vi "DefendAreaTacticVSS.vi"(7 "First call?":bool=TRUE, 8 "error in (no error)":errorcluster, 9 "Game in":refnum<class "Game.lvclass">, 10 "Robot":refnum<class "Robot.lvclass">, 11 "DefendAreaTacticVSS in":refnum<class "DefendAreaTacticVSS.lvclass">) -> (0 "error out":errorcluster, 2 "Robot out":refnum<class "Robot.lvclass">, 3 "DefendAreaTacticVSS out":refnum<class "DefendAreaTacticVSS.lvclass">)   [LabVIEW 2020, in "DefendAreaTacticVSS.lvclass"]
uses:
  DefendAreaTacticVSS.lvclass
  Robot_class/Robot.lvclass
  Game_class/Game.lvclass
  Robot_class/tactics.ctl
  Tactic_class/Tactic.lvclass/Tactic.ctl
  Robot_class/Robot.lvclass/Robot.ctl
  Tactic_class/Read Skillbook.vi
  Robot_class/Write tactic.vi
  Skillbook_class/Skillbook.lvclass
  KickSkillVSS_class/KickSkillVSS.lvclass
  PenaltyPosSkillVSS_class/PenaltyPosSkillVSS.lvclass
  BallDispPosSkillVSS_class/BallDispPosSkillVSS.lvclass
  BallToGoalSkillVSS_class/BallToGoalSkillVSS.lvclass
  GoToBallSkillVSS_class/GoToBallSkillVSS.lvclass
  DefBallPosSkillVSS_class/DefBallPosSkillVSS.lvclass
  HaltSkill_class/HaltSkill.lvclass
panel:
  out "x .or. y?":bool
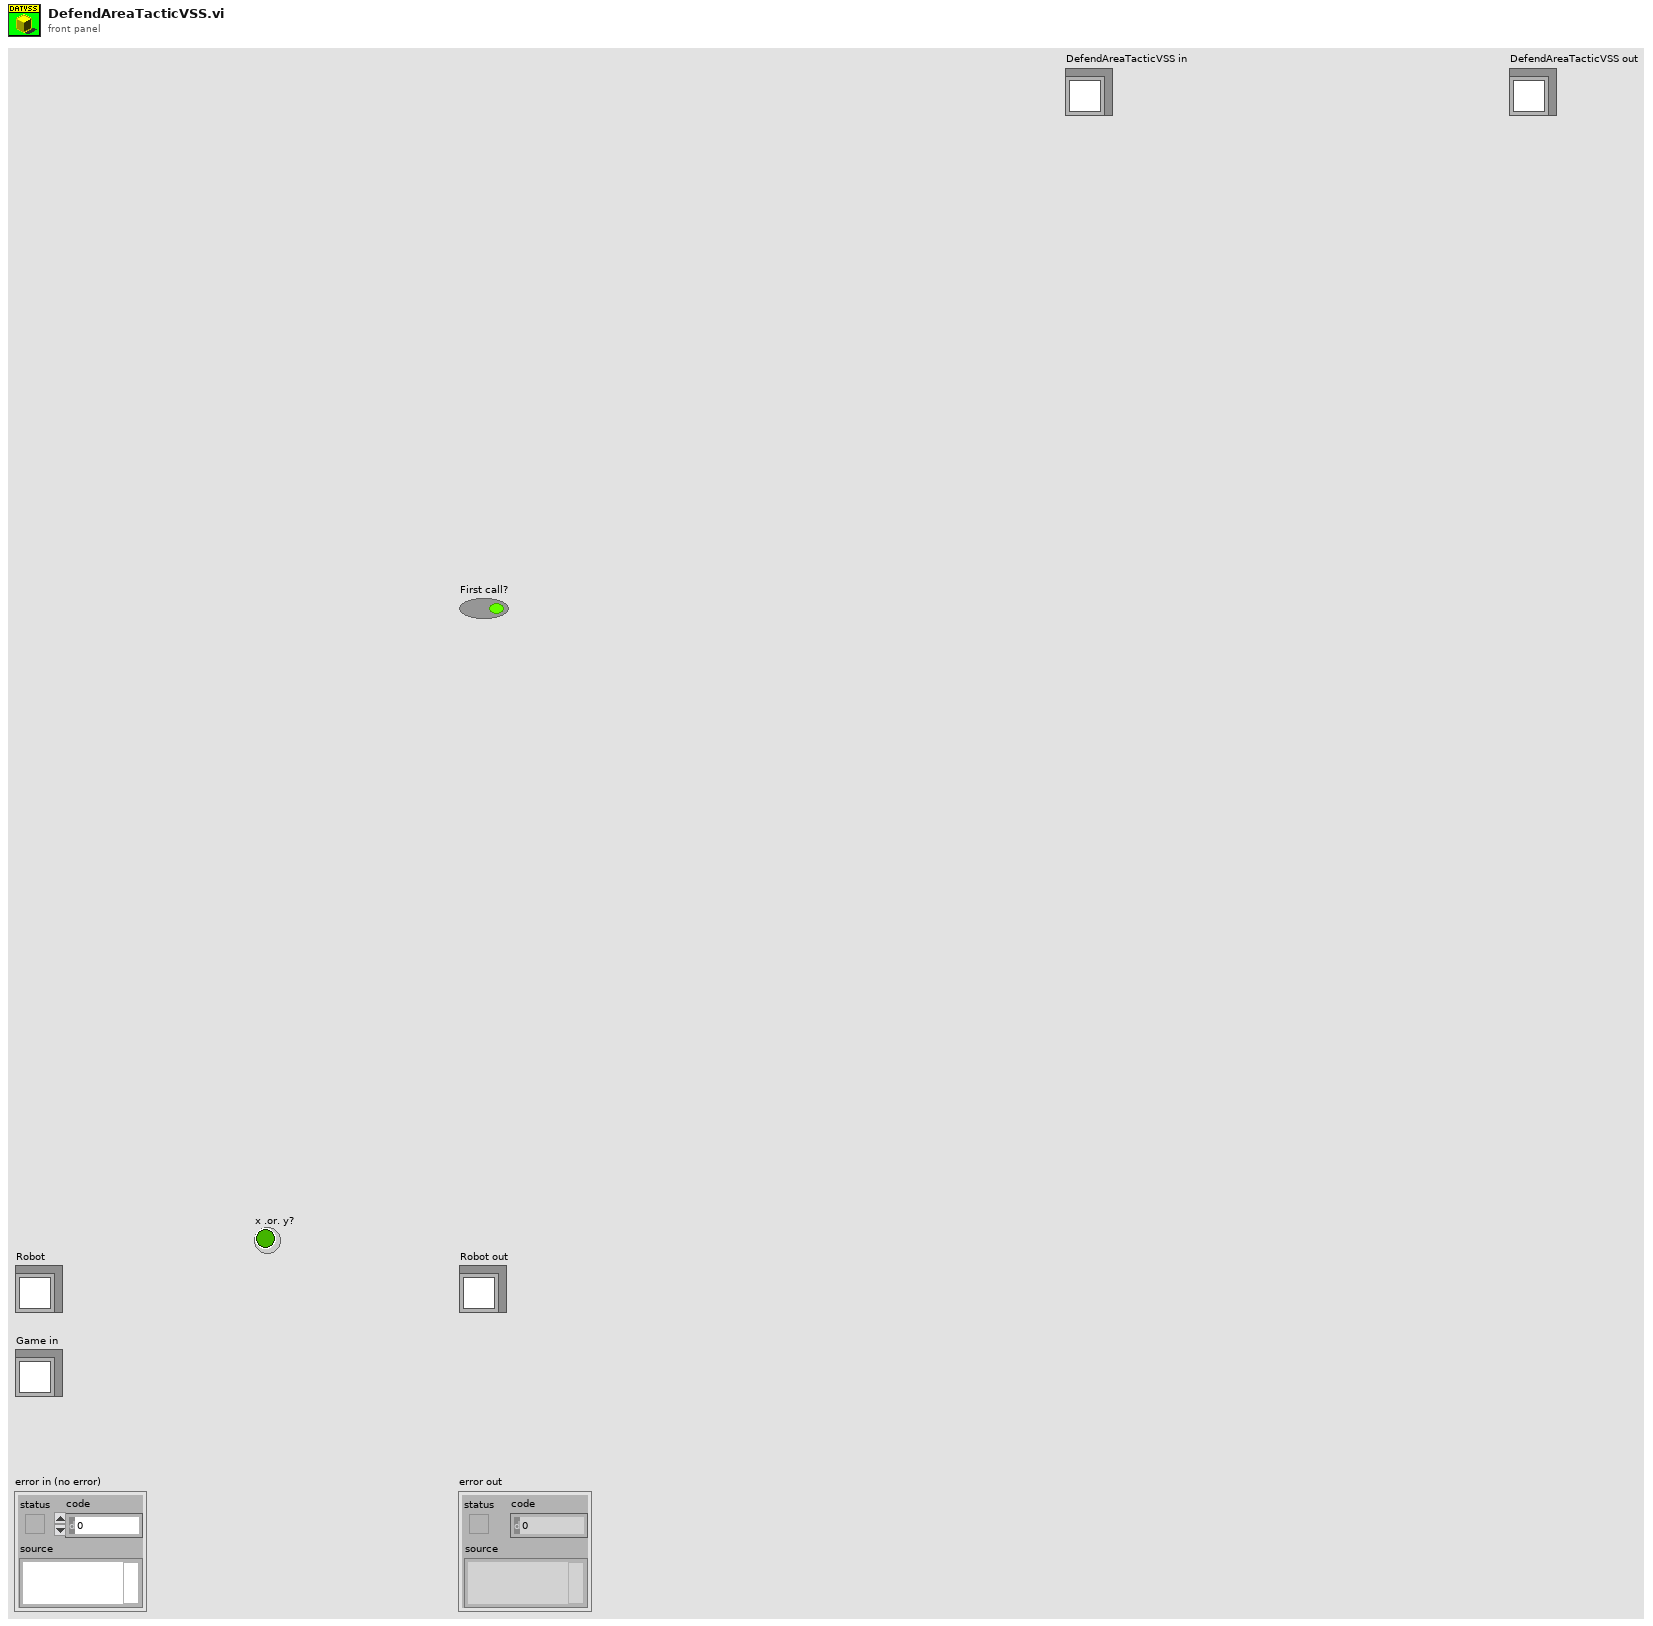
[diagram p1: front panel]
types:
  T1 = typedef "tactics.ctl" = enum16{"ReceivePassInFuturePoint", "Roller", "PrepareRollToPassRollerGoTo", "PrepareRollToPassReceiverGoTo", "WaitRoll", "PositionToRoll", "PenaltyAttacker", "PassObserver", "PenaltyDefense", "TableReceiverTactic", "Test", "DefendGoal", "Marker", "FollowAttacker", "DefendArea", "Shoot", "AttackerAimGoal", "AttackerBallOutOfField", "AttackerBlock", "AttackerStop", "Duelist", "Halt", "ZigZag", "GoTo", "Timeout", "KickToPassReceiver", "PositionToReceivePass", "DefendAreaVSS", "DefendGoalVSS", "KickVSS", "AttackVSS", "DispBallVSS", "PenaltyAttackVSS", "WaitPass"}
  T2 = cluster{"KickSkillVSS":refnum<class "KickSkillVSS.lvclass">, "PenaltyPosSkillVSS":refnum<class "PenaltyPosSkillVSS.lvclass">, "BallDispPosSkillVSS":refnum<class "BallDispPosSkillVSS.lvclass">, "BallToGoalSkillVSS":refnum<class "BallToGoalSkillVSS.lvclass">, "GoToBallSkillVSS":refnum<class "GoToBallSkillVSS.lvclass">, "DefBallPosSkillVSS":refnum<class "DefBallPosSkillVSS.lvclass">, "HaltSkill":refnum<class "HaltSkill.lvclass">}
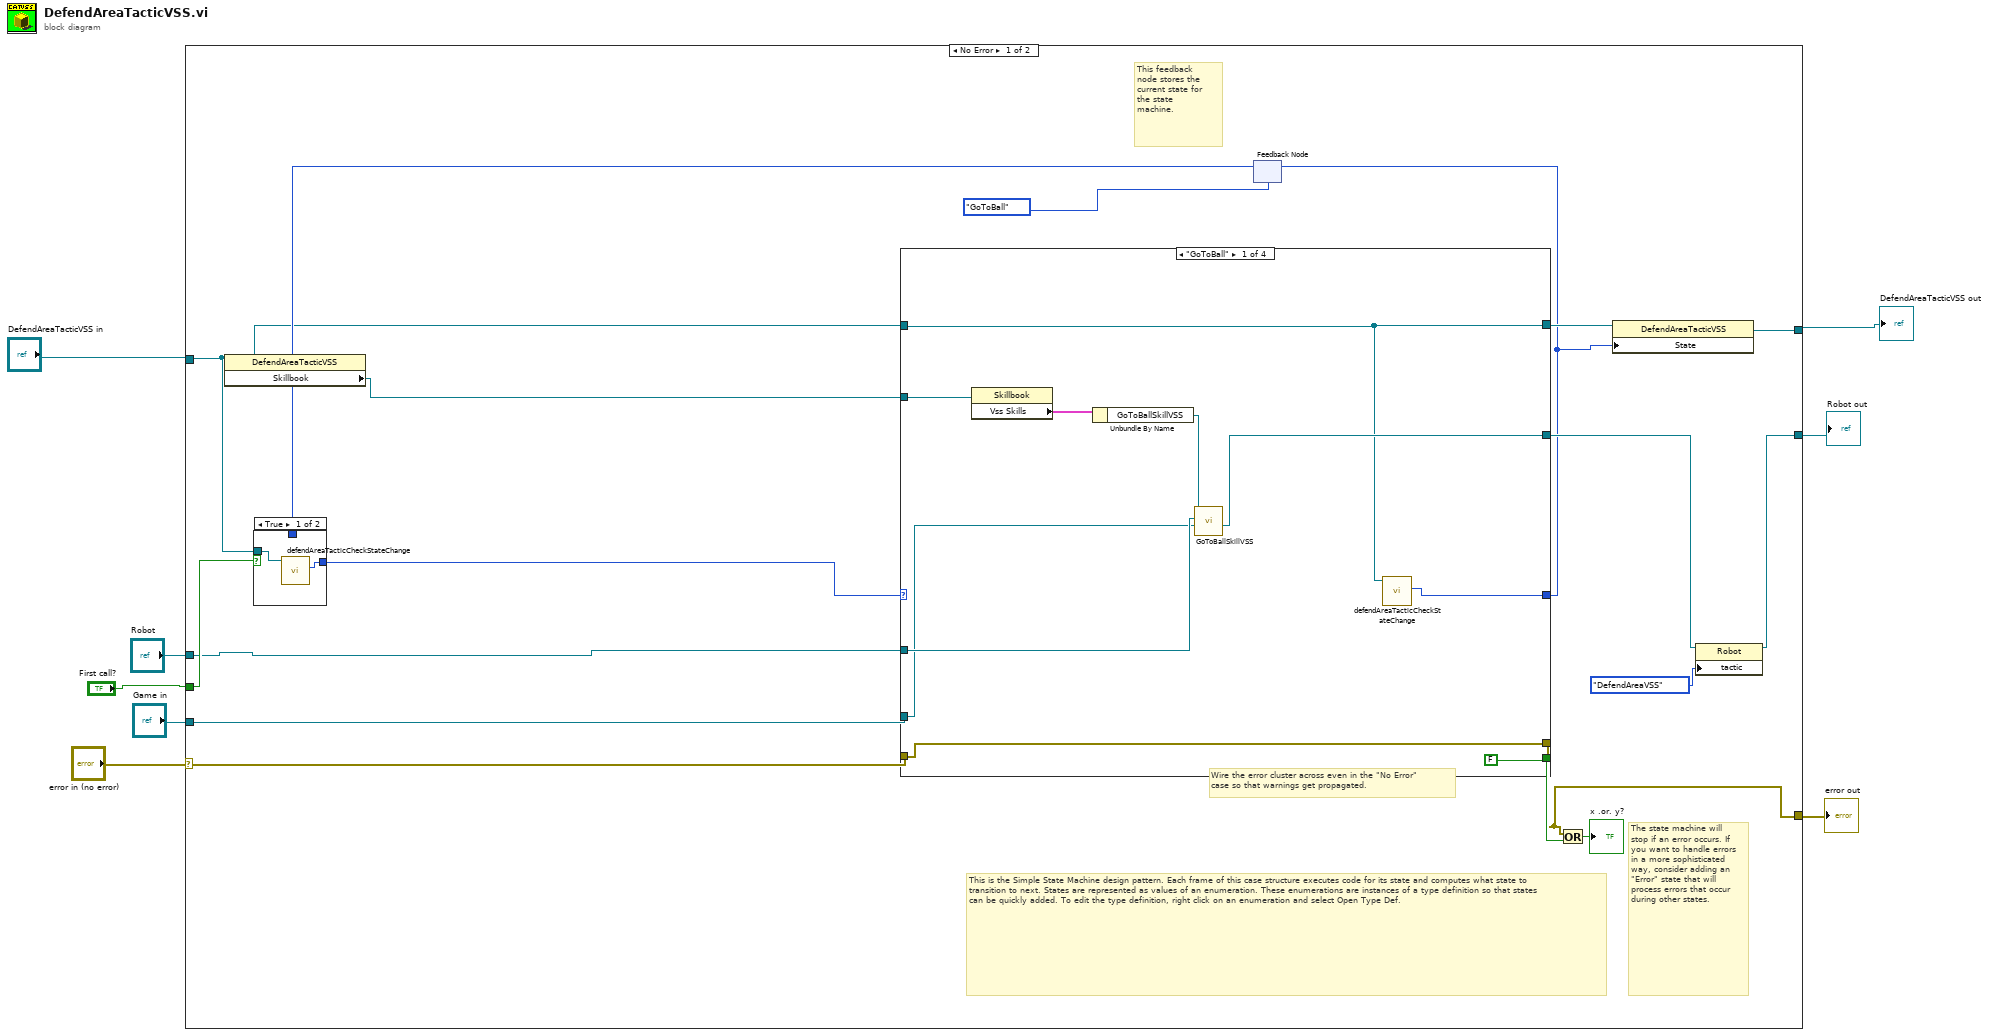
[diagram p0: block diagram]
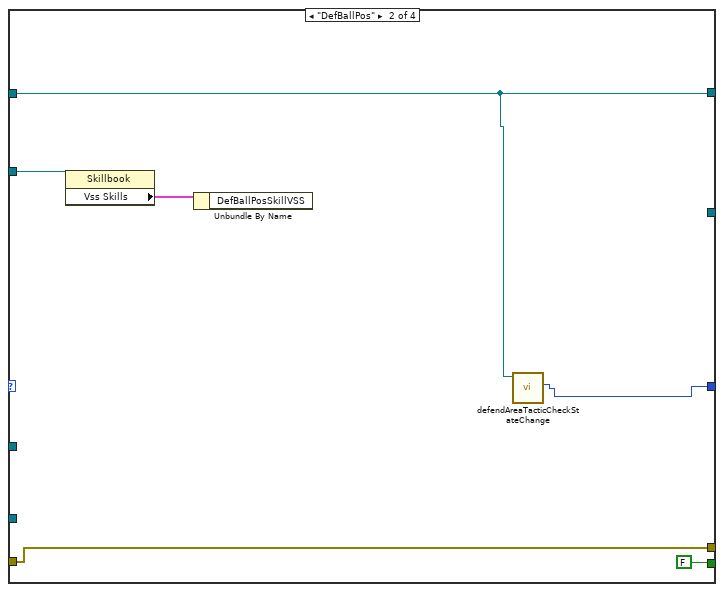
[diagram p3: hidden frame]
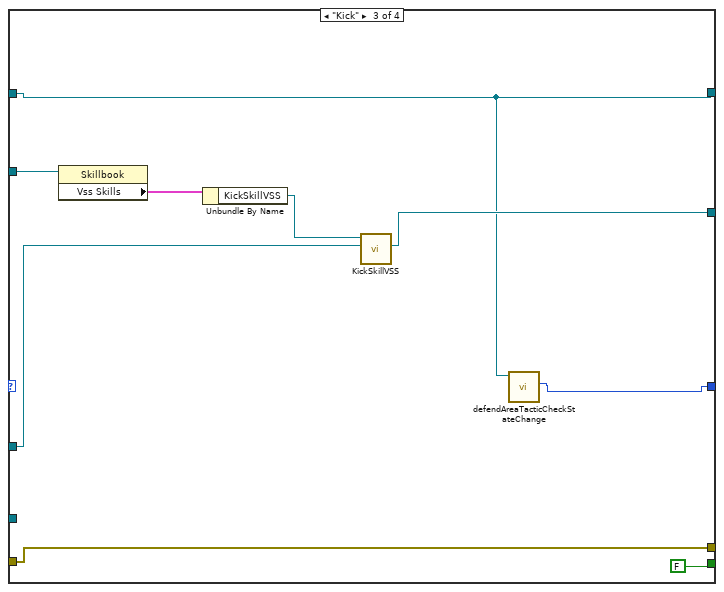
[diagram p4: hidden frame]
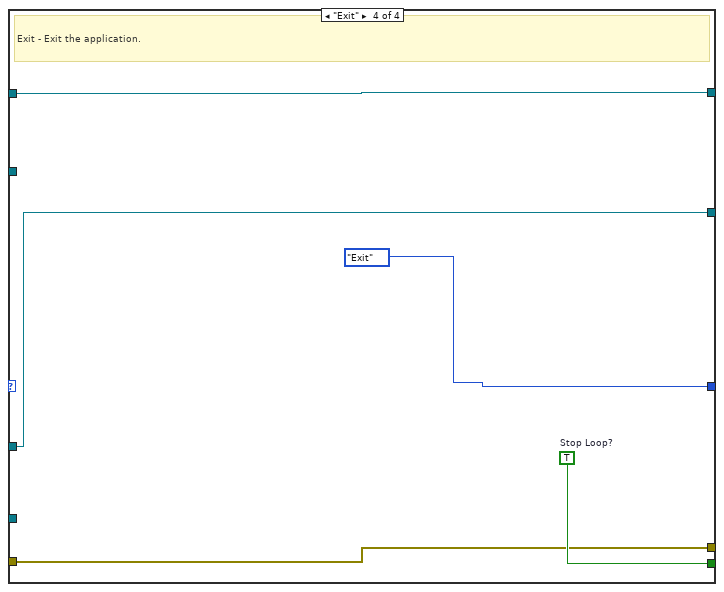
[diagram p5: hidden frame]
diagram:
  n1 = case shown="No Error" "error in (no error)" {
    selector: "error in (no error)" -> [w22 w62]
    tunnel: [w21 w62] -> w7
    tunnel: [w20 w61] -> w1
    tunnel: "DefendAreaTacticVSS in" -> [w12 w61]
    tunnel: "Robot" -> [w10 w60]
    tunnel: "Game in" -> [w16 _]
    tunnel: [w17 w60] -> w4
    tunnel: "First call?" -> [w15 _]
    frame No Error {
      # "The state machine will stop if an error occurs. If you want to handle errors in a more sophisticated way, consider adding an \"Error\" state that will process errors that occur during other states."
      # "This feedback node stores the current state for the state machine."
      # "This is the Simple State Machine design pattern. Each frame of this case structure executes code for its state and computes what state to transition to next. States are represented as values of an enumeration. These enumerations are instances of a type definition so that states can be quickly added. To edit the type definition, right click on an enumeration and select Open Type Def."
      # "Wire the error cluster across even in the \"No Error\"\ncase so that warnings get propagated."
      n2 = property class="DefendAreaTacticVSS"(reference=w12) -> ("Skillbook"=w24:refnum<class "Skillbook.lvclass">)  [unwired: 1 in, 2 out]
      n3 = feedback #1(enum16{"Exit", "Kick", "DefBallPos", "GoToBall"}."GoToBall" ("State")) -> (w14:enum16{"Exit", "Kick", "DefBallPos", "GoToBall"})
      n4 = case shown="True" w15 {
        tunnel: [w27 w29] -> w13
        tunnel: w14 -> [_ w29]
        tunnel: w12 -> [w28 _]
        frame True {
          n5 = call "defendAreaTacticCheckStateChange.vi"("DefendAreaTacticVSS in"=w28) -> ("State"=w27:enum16{"Exit", "Kick", "DefBallPos", "GoToBall"})  [unwired: 8 in, 2 out]
        }
        frame False {
        }
      }
      n6 = case shown="\"GoToBall\"" w13 {
        tunnel: [w35 w40 w46 enum16{"Exit", "Kick", "DefBallPos", "GoToBall"}."Exit" ("State")] -> w11
        tunnel: [FALSE FALSE FALSE w59] -> w26
        tunnel: w24 -> [w38 w44 w53 _]
        tunnel: w10 -> [w32 _ w49 w58]
        tunnel: [w34 _ w48 w58] -> w18
        tunnel: [w33 w41 w47 w57] -> w23
        tunnel: w12 -> [w33 w41 w47 w57]
        tunnel: w16 -> [w31 _ _ _]
        tunnel: [w37 w43 w51 w56] -> w21
        tunnel: w22 -> [w37 w43 w51 w56]
        frame "GoToBall" {
          n7 = property class="Skillbook"(reference=w38) -> ("Vss Skills"=w39:T2)  [unwired: 1 in, 2 out]
          n8 = Unbundle By Name(w39) -> ("GoToBallSkillVSS"=w30:refnum<class "GoToBallSkillVSS.lvclass">)
          n9 = call "GoToBallSkillVSS.vi"("Game"=w31, "Robot in"=w32, "GoToBallSkillVSS in"=w30) -> ("Robot out"=w34:refnum<class "Robot.lvclass">)  [unwired: 6 in, 2 out]
          n10 = call "defendAreaTacticCheckStateChange.vi"("DefendAreaTacticVSS in"=w33) -> ("State"=w35:enum16{"Exit", "Kick", "DefBallPos", "GoToBall"})  [unwired: 8 in, 2 out]
        }
        frame "DefBallPos" {
          n11 = property class="Skillbook"(reference=w44) -> ("Vss Skills"=w45:T2)  [unwired: 1 in, 2 out]
          n12 = Unbundle By Name(w45) -> ()  [unwired: 1 out]
          n13 = call "defendAreaTacticCheckStateChange.vi"("DefendAreaTacticVSS in"=w41) -> ("State"=w40:enum16{"Exit", "Kick", "DefBallPos", "GoToBall"})  [unwired: 8 in, 2 out]
        }
        frame "Kick" {
          n14 = property class="Skillbook"(reference=w53) -> ("Vss Skills"=w54:T2)  [unwired: 1 in, 2 out]
          n15 = Unbundle By Name(w54) -> ("KickSkillVSS"=w50:refnum<class "KickSkillVSS.lvclass">)
          n16 = call-dynamic "KickSkillVSS.vi"("Robot"=w49, "KickSkillVSS in"=w50) -> ("Robot out"=w48:refnum<class "Robot.lvclass">)  [unwired: 7 in, 2 out]
          n17 = call "defendAreaTacticCheckStateChange.vi"("DefendAreaTacticVSS in"=w47) -> ("State"=w46:enum16{"Exit", "Kick", "DefBallPos", "GoToBall"})  [unwired: 8 in, 2 out]
        }
        frame "Exit" {
          w59 = TRUE  # Stop Loop?
          # "Exit - Exit the application."
        }
      }
      n18 = feedback-in #1(w11) -> ()
      n19 = Or(x=w21, y=w26) -> (x .or. y?=→"x .or. y?":bool)
      n20 = property class="DefendAreaTacticVSS"(reference=w23, "State"=w11) -> (reference out=w20:refnum<class "DefendAreaTacticVSS.lvclass">)  [unwired: 1 in, 1 out]
      n21 = property class="Robot"(reference=w18, "tactic"=tactics."DefendAreaVSS") -> (reference out=w17:refnum<class "Robot.lvclass">)  [unwired: 1 in, 1 out]
    }
    frame Error {
    }
  }
  "DefendAreaTacticVSS out" <- w1
  "error out" <- w7
  "Robot out" <- w4
